vi "Tektronix MSO5X Test_2018.vi"() -> ()   [LabVIEW 2018]
doc: "Demonstrates how to set up an oscilloscope automatically. You can configure this VI to acquire waveforms continuously from a single channel by following the following steps:\n\n1. Specify a valid VISA resource to use. \n2. Specify a channel. \n3. Specify a time-out value for reading a waveform.\n4. Specifies the start and end point for reading a waveform.\n5. Run this VI. The <B>Waveform Graph</B> displays the waveform you acquire."
uses:
  C/Program Files (x86)/National Instruments/LabVIEW 2019/instr.lib/Tektronix MSO5X Series/Tektronix MSO5X Series.lvlib
  C/Program Files (x86)/National Instruments/LabVIEW 2019/instr.lib/Tektronix MSO5X Series/Public/Data/Read (Single Waveform).vi
panel:
  out "Waveform Graph":waveform(dbl)(graph)
  in  "Close Button":bool
  in  "Channel (CH1)":string="CH1"
  in  "Ref Waveform Type":u16(ring) items=["Normal", "Came from a MATH"]
  in  "Ending Point (2500)":i32=2500
  in  "Starting Point (1)":i32=1
  in  "Net Attenuation (1.0)":dbl=1.0
  in  "Maximum Time (100000 ms)":u32=100000
  in  "VISA resource name":refnum<visa-resource-name>
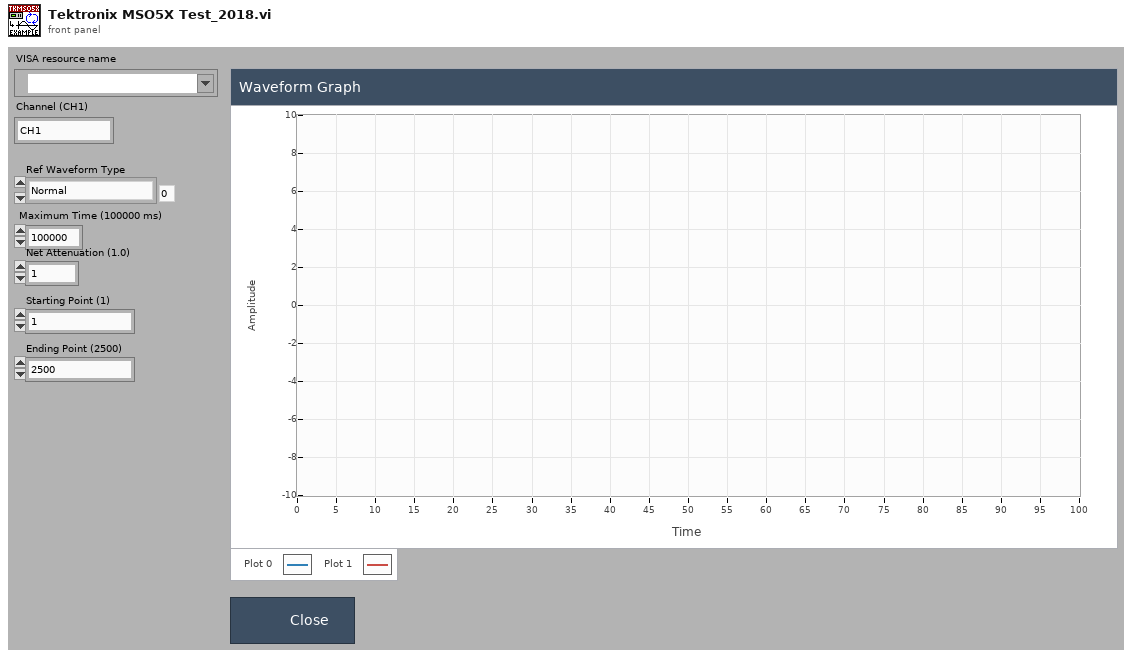
[diagram p1: front panel]
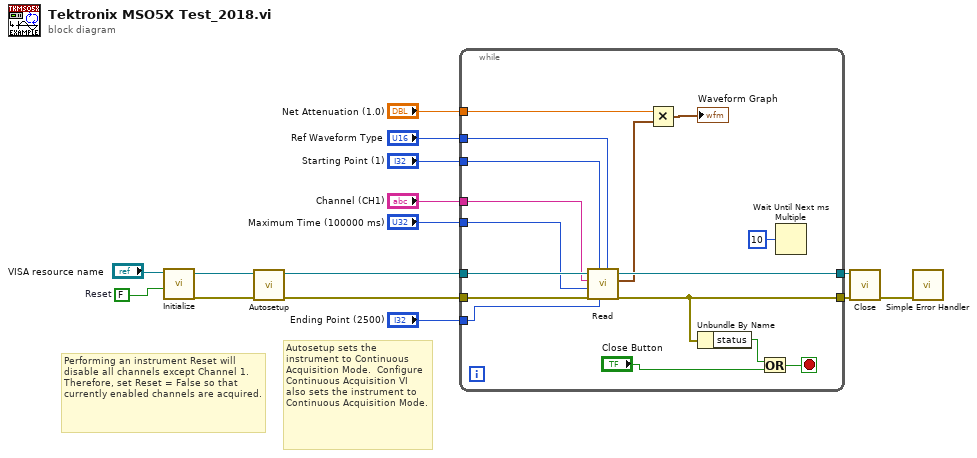
[diagram p0: block diagram]
diagram:
  w6 = FALSE  # Reset
  # "Performing an instrument Reset will disable all channels except Channel 1. Therefore, set Reset = False so that currently enabled channels are acquired."
  # "Autosetup sets the instrument to Continuous Acquisition Mode.  Configure Continuous Acquisition VI also sets the instrument to Continuous Acquisition Mode."
  n1 = call "Initialize.vi"("Reset (True)"=w6, "VISA resource name"="VISA resource name") -> ("error out"=w10:errorcluster, "VISA resource name out"=w11:refnum<visa-resource-name>)  [unwired: 8 in]
  n2 = call "Autosetup.vi"("error in (no error)"=w10, "VISA resource name"=w11) -> ("error out"=w8:errorcluster, "VISA resource name out"=w9:refnum<visa-resource-name>)  [unwired: 8 in]
  n3 = while {
    tunnel: w9 -> [w26]
    tunnel: w8 -> [w25]
    tunnel: [w27] -> w15
    tunnel: [w28] -> w14
    tunnel: "Maximum Time (100000 ms)" -> [w23]
    tunnel: "Net Attenuation (1.0)" -> [w22]
    tunnel: "Starting Point (1)" -> [w21]
    tunnel: "Ending Point (2500)" -> [w20]
    tunnel: "Ref Waveform Type" -> [w19]
    tunnel: "Channel (CH1)" -> [w18]
    stop <- w29 stop-if-true
    n4 = call-poly "Read.vi"("Ref Waveform Type"=w19, "Ending Point (2500)"=w20, "Starting Point (1)"=w21, "error in (no error)"=w25, "Maximum Time (100000 ms)"=w23, "Channel (CH1)"=w18, "VISA resource name"=w26) -> ("error out"=w28:errorcluster, "Waveform Graph"=w24:waveform(dbl), "VISA resource name out"=w27:refnum<visa-resource-name>)  [unwired: 2 in]
    n5 = Multiply(x=w22, y=w24) -> (x*y=→"Waveform Graph":waveform(dbl))
    n6 = Unbundle By Name(w28) -> ("status"=w30:bool)
    n7 = Or(x=w30, y="Close Button") -> (x .or. y?=w29:bool)
    n8 = Wait Until Next ms Multiple(millisecond multiple=u32 10) -> ()  [unwired: 1 out]
  }
  n9 = call "Close.vi"("error in (no error)"=w14, "VISA resource name"=w15) -> ("error out"=w13:errorcluster)  [unwired: 9 in]
  n10 = call <vilib>:"Simple Error Handler.vi"("error in (no error)"=w13) -> ()  [unwired: 4 in, 5 out]
